vi "stabilizePress_04.vi"() -> ()   [LabVIEW 2011]
uses:
  <vilib>/Platform/TimedLoop/XDataNode/timing_clust.ctl
  <vilib>/Platform/TimedLoop/XDataNode/nitl_modes.ctl
  <vilib>/Platform/TimedLoop/XDataNode/wakeup.ctl
  <vilib>/Platform/TimedLoop/XDataNode/XDataNode.xnode
  <vilib>/Platform/TimedLoop/XDataNode/XDNodeRunTimeDep.lvlib
panel:
  out "tElaps":dbl
  in  "dT_fit(s)":dbl=20.0
  in  "tTotal(s)":dbl=20.0
  out "tNow":dbl
  out "XY Graph":cluster{"Value":dbl[], "Value":dbl[]}(graph)
  out "tune Setpoint(torr)":dbl=20.0
  in  "t array":dbl[](array[numeric])=[1.0, 2.0, 3.0, 4.0, 5.0, 6.0, 7.0, 8.001, 9.0, 10.0, 11.0, 12.0, 13.0, 14.0, 15.0, 16.0, 17.0, 18.001, 19.0, 20.0, 21.0, 22.0]
  out "P array":dbl[](array[numeric])=[20.39, 19.689999999999998, 19.299999999999997, 19.189999999999998, 19.130000000000003, 19.110000000000003, 19.09, 19.08, 19.07, 19.05, 19.04, 19.04, 19.05, 19.05, 19.05, 19.04, 19.05, 19.060000000000002, 19.060000000000002, 19.05, 19.05, 19.05]
  out "stabilize done":bool=TRUE
  in  "tExp(s)":dbl=20.0
  out "Set Point (torr)":dbl=20.0 format="%.2f"
  out "Setpoint Index":string="C"
  out "Setpoint Index control":u16(ring)=2 caption="Setpoint" items=["A", "B", "C", "D"]
  out "first":bool
  out "tStart":dbl=22.0
  in  "time done (s)":dbl
  out "Wait to set":bool
  out "IO error":errorcluster
  in  "stop":bool
  out "P (torr)":dbl=19.05 format="%.2f"
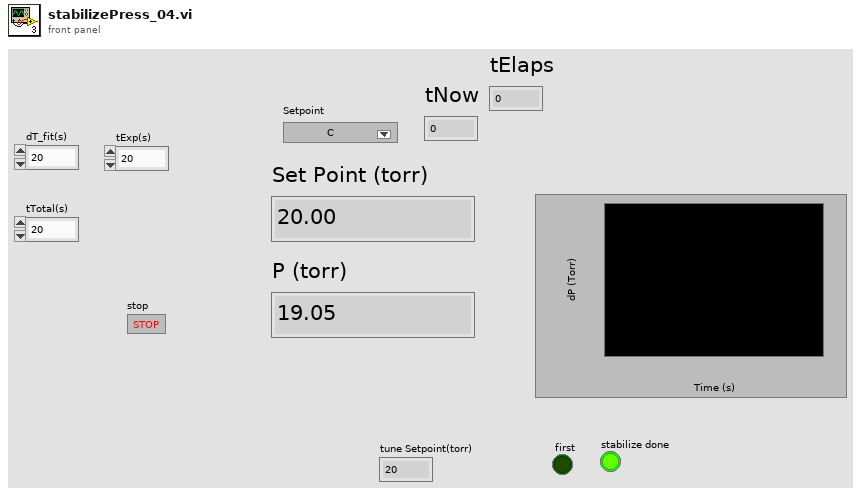
[diagram p1: front panel]
types:
  T1 = typedef "XDNodeRunTimeDep.lvlib/timing_clust.ctl" = cluster{"Expected End [f-1]":u64, "Actual End [f-1]":u64, "Finished Late? [f-1]":bool, "Expected End [i-1]":u64, "Actual End [i-1]":u64, "Finished Late? [i-1]":bool, "Expected Start [i]":u64, "Actual Start [i]":u64, "Expected Start [f]":u64, "Actual Start [f]":u64, "Source Name":string, "Structure Name":string, "Period":i64, "Deadline":i64, "Offset":i64, "Start":i64, "Priority":i32, "Timeout":i32, "Mode":T2, "Wakeup Reason":T3, "Error":errorcluster, "Source Type":string, "Secondary Source Type":string, "Global End Time":u64, "Global Start Time":u64, "Frame Duration":u64, "Iteration Duration":u64, "Assigned CPU":i32, "I/O Scan Engine Mode":u32}
  T2 = typedef "XDNodeRunTimeDep.lvlib/nitl_modes.ctl" = enum32{"No Change", "Process missed periods, maintain original phase", "Discard missed periods, maintain original phase", "Process missed periods, ignore original phase", "Discard missed periods, ignore original phase"}
  T3 = typedef "XDNodeRunTimeDep.lvlib/wakeup.ctl" = enum32{"Normal", "Aborted", "Asynchronous wakeup", "Timing source error", "Timed loop error", "Timeout"}
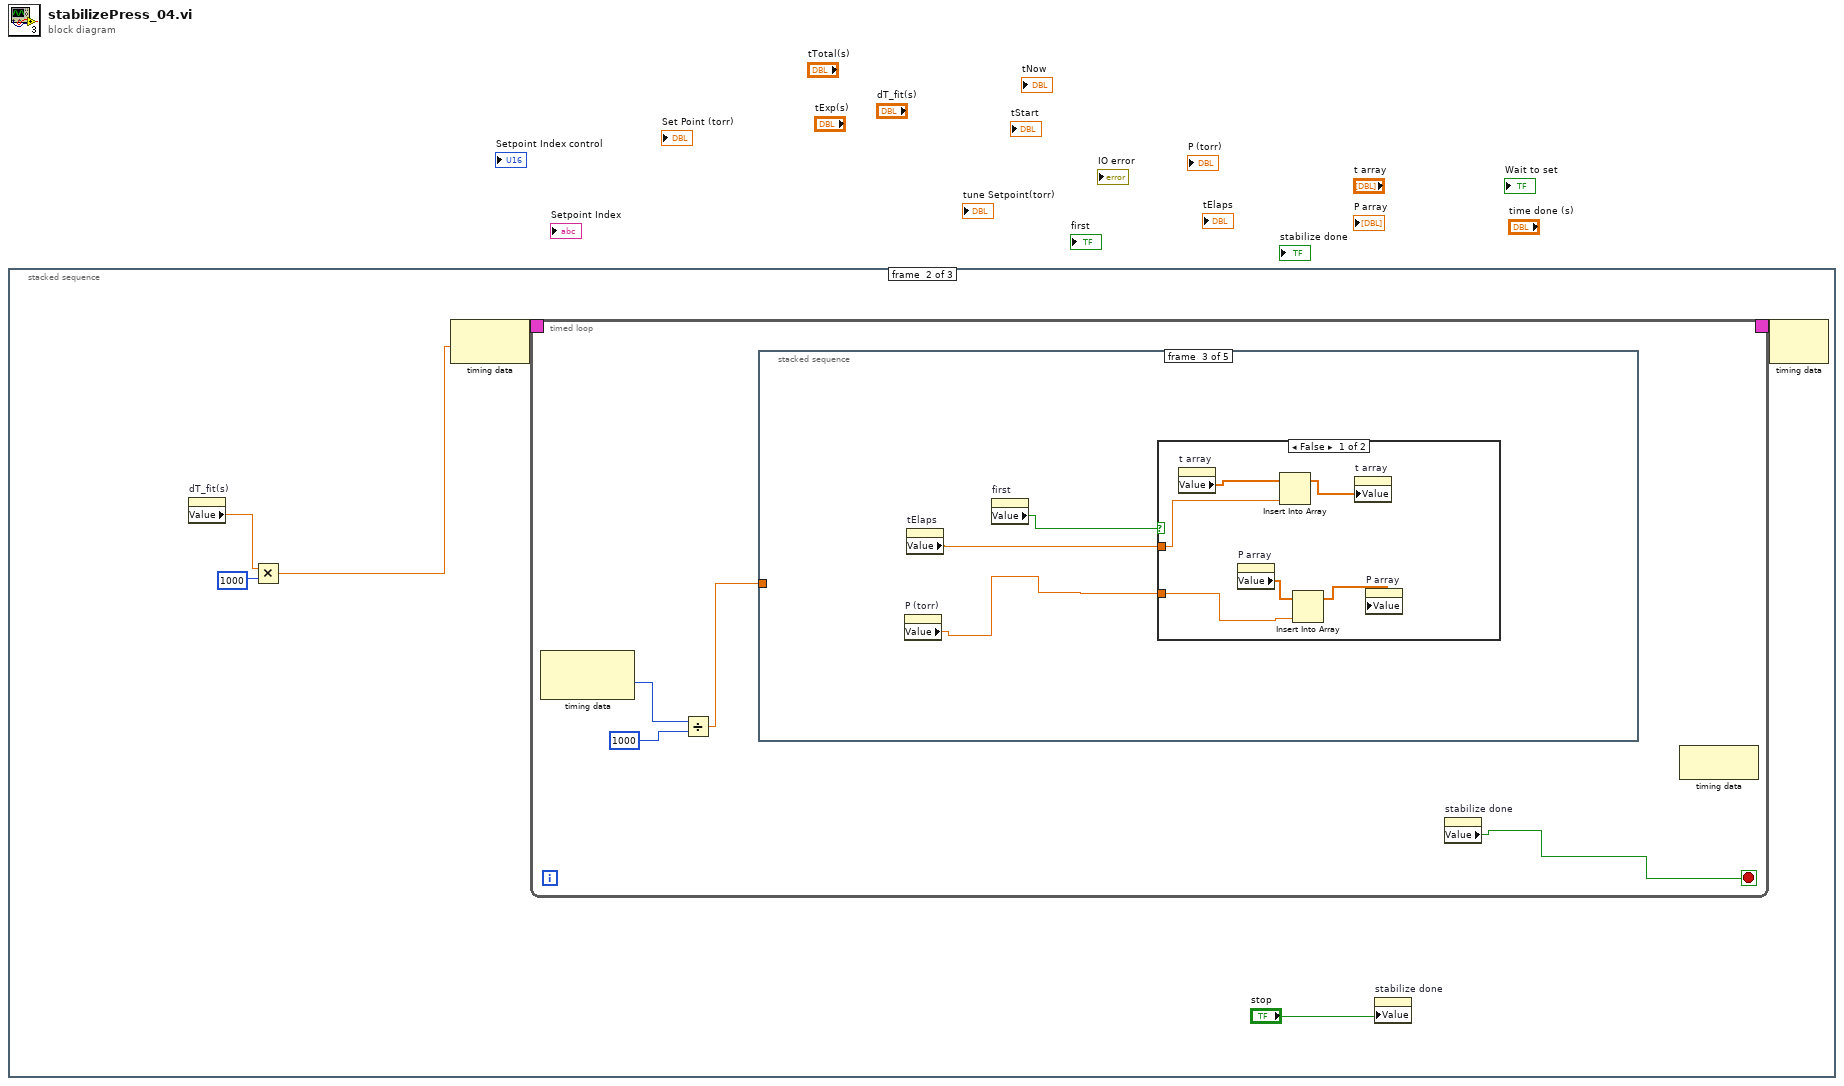
[diagram p0: block diagram]
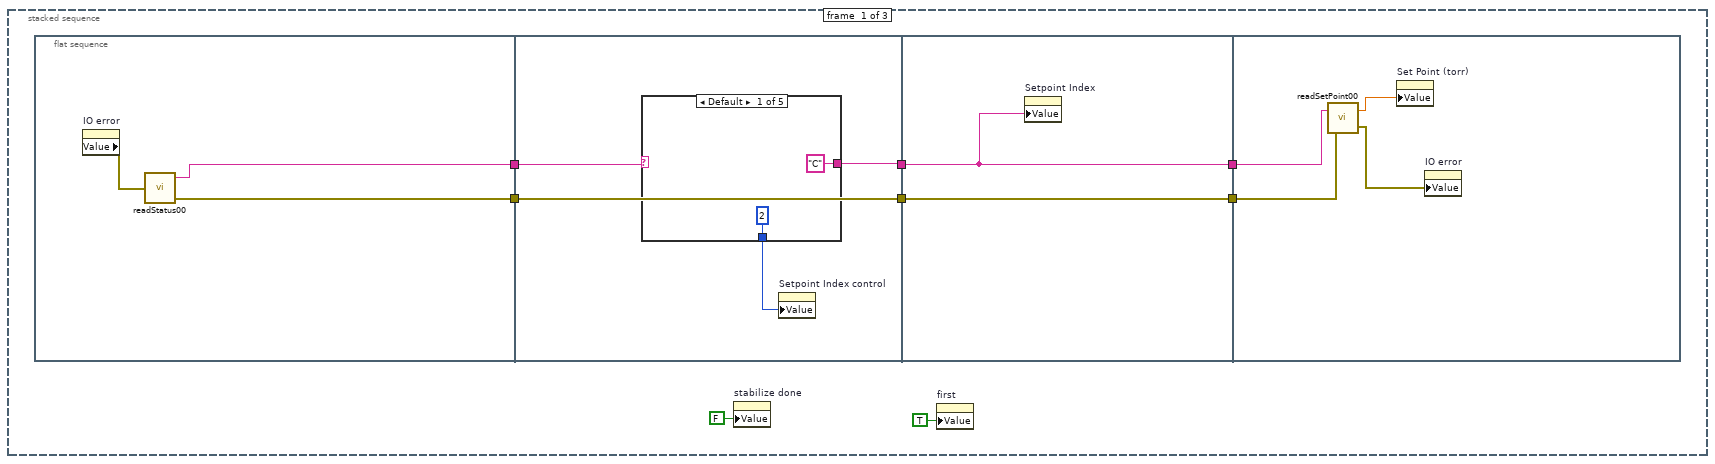
[diagram p2: hidden frame]
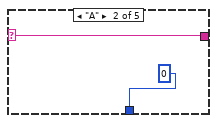
[diagram p3: hidden frame]
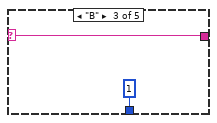
[diagram p4: hidden frame]
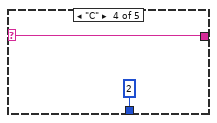
[diagram p5: hidden frame]
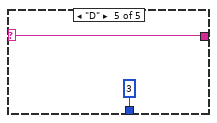
[diagram p6: hidden frame]
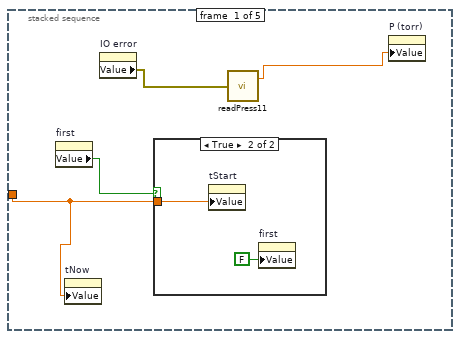
[diagram p7: hidden frame]
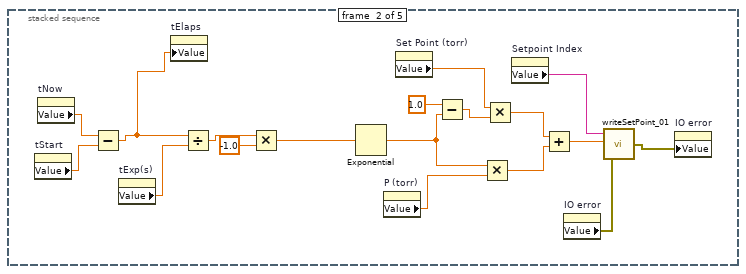
[diagram p9: hidden frame]
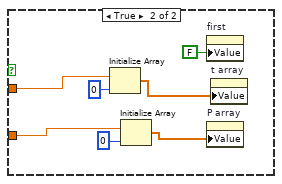
[diagram p10: hidden frame]
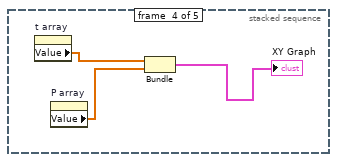
[diagram p11: hidden frame]
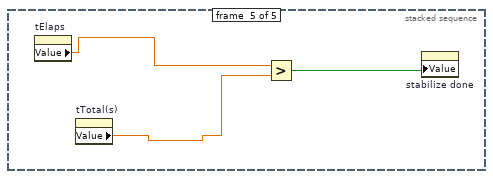
[diagram p12: hidden frame]
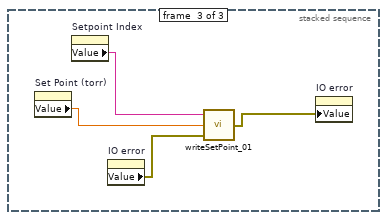
[diagram p13: hidden frame]
diagram:
  n1 = stacked-sequence {
    frame #0 {
      n2 = flat-sequence {
        tunnel: [w10] -> w8
        tunnel: [w9] -> w7
        tunnel: w8 -> [w14]
        tunnel: [w13] -> w6
        tunnel: w7 -> [w15]
        tunnel: [w15] -> w5
        tunnel: w6 -> [w26]
        tunnel: [w26] -> w4
        tunnel: w5 -> [w27]
        tunnel: [w27] -> w3
        tunnel: w4 -> [w31]
        tunnel: w3 -> [w30]
        frame #0 {
          n3 = property on="IO error" class="Clust (strict)"() -> ("Value"=w11:errorcluster)  [unwired: 2 in, 2 out]
          n4 = call "readStatus00.vi"("error in"=w11) -> ("Setpoint"=w10:string, "error out"=w9:errorcluster)  [unwired: 1 out]
        }
        frame #1 {
          n5 = case shown="Default" w14 {
            selector: w14 -> [_ w19 w20 w22 w24]
            tunnel: ["C" w19 w20 w22 w24] -> w13
            tunnel: [u16 2 ("Ring") u16 0 ("Ring") u16 1 ("Ring") u16 2 ("Ring") u16 3 ("Ring")] -> w12
            frame Default {
            }
            frame "A" {
            }
            frame "B" {
            }
            frame "C" {
            }
            frame "D" {
            }
          }
          n6 = property on="Setpoint Index control" class="Ring (strict)"("Value"=w12) -> ()  [unwired: 2 in, 2 out]
        }
        frame #2 {
          n7 = property on="Setpoint Index" class="Str"("Value"=w26) -> ()  [unwired: 2 in, 2 out]
        }
        frame #3 {
          n8 = call "readSetPoint00.vi"("error in"=w30, "Setpoint"=w31) -> ("error out"=w29:errorcluster, "P"=w28:dbl)
          n9 = property on="Set Point (torr)" class="DigNum (strict)"("Value"=w28) -> ()  [unwired: 2 in, 2 out]
          n10 = property on="IO error" class="Clust (strict)"("Value"=w29) -> ()  [unwired: 2 in, 2 out]
        }
      }
      n11 = property on="stabilize done" class="Bool (strict)"("Value"=FALSE ("fit done")) -> ()  [unwired: 2 in, 2 out]
      n12 = property on="first" class="Bool (strict)"("Value"=TRUE ("first")) -> ()  [unwired: 2 in, 2 out]
    }
    frame #1 {
      n13 = property on="dT_fit(s)" class="DigNum (strict)"() -> ("Value"=w33:dbl)  [unwired: 2 in, 2 out]
      n14 = Multiply(x=w33, y=u32 1000) -> (x*y=w34:dbl)
      n15 = node-c288(w34) -> (w37:T1)
      n16 = timed-loop {
        timing: w37 -> [_]
        timing-out: [_] -> w36
        stop <- w38 stop-if-true
        n17 = node-c288() -> (w41:i64)  [unwired: 1 in, 1 out]
        n18 = Divide(x=w41, y=i64 1000) -> (x/y=w39:dbl)
        n19 = stacked-sequence {
          tunnel: w39 -> [w42 _ _ _ _]
          frame #0 {
            n20 = property on="first" class="Bool (strict)"() -> ("Value"=w44:bool)  [unwired: 2 in, 2 out]
            n21 = property on="tNow" class="DigNum (strict)"("Value"=w42) -> ()  [unwired: 2 in, 2 out]
            n22 = property on="IO error" class="Clust (strict)"() -> ("Value"=w45:errorcluster)  [unwired: 2 in, 2 out]
            n23 = case shown="True" w44 {
              tunnel: w42 -> [_ w47]
              frame False {
              }
              frame True {
                n24 = property on="tStart" class="DigNum (strict)"("Value"=w47) -> ()  [unwired: 2 in, 2 out]
                n25 = property on="first" class="Bool (strict)"("Value"=FALSE ("first")) -> ()  [unwired: 2 in, 2 out]
              }
            }
            n26 = call "readPress11.vi"("error in"=w45) -> ("P"=w43:dbl)  [unwired: 1 out]
            n27 = property on="P (torr)" class="DigNum (strict)"("Value"=w43) -> ()  [unwired: 2 in, 2 out]
          }
          frame #1 {
            n28 = property on="tStart" class="DigNum (strict)"() -> ("Value"=w64:dbl)  [unwired: 2 in, 2 out]
            n29 = property on="tNow" class="DigNum (strict)"() -> ("Value"=w65:dbl)  [unwired: 2 in, 2 out]
            n30 = Subtract(x=w65, y=w64) -> (x-y=w48:dbl)
            n31 = property on="tExp(s)" class="DigNum (strict)"() -> ("Value"=w63:dbl)  [unwired: 2 in, 2 out]
            n32 = property on="tElaps" class="DigNum (strict)"("Value"=w48) -> ()  [unwired: 2 in, 2 out]
            n33 = Divide(x=w48, y=w63) -> (x/y=w62:dbl)
            n34 = Multiply(x=w62, y=-1.0) -> (x*y=w60:dbl)
            n35 = Exponential(1:w60) -> (0:w55:dbl)
            n36 = property on="P (torr)" class="DigNum (strict)"() -> ("Value"=w56:dbl)  [unwired: 2 in, 2 out]
            n37 = property on="Set Point (torr)" class="DigNum (strict)"() -> ("Value"=w57:dbl)  [unwired: 2 in, 2 out]
            n38 = Subtract(x=1.0, y=w55) -> (x-y=w58:dbl)
            n39 = Multiply(x=w55, y=w56) -> (x*y=w53:dbl)
            n40 = Multiply(x=w57, y=w58) -> (x*y=w54:dbl)
            n41 = property on="Setpoint Index" class="Str"() -> ("Value"=w51:string)  [unwired: 2 in, 2 out]
            n42 = Add(x=w54, y=w53) -> (x+y=w52:dbl)
            n43 = property on="IO error" class="Clust (strict)"() -> ("Value"=w50:errorcluster)  [unwired: 2 in, 2 out]
            n44 = call "writeSetPoint_01.vi"("error in"=w50, "P (Torr)"=w52, "Setpoint"=w51) -> ("error out"=w49:errorcluster)
            n45 = property on="IO error" class="Clust (strict)"("Value"=w49) -> ()  [unwired: 2 in, 2 out]
          }
          frame #2 {
            n46 = property on="P (torr)" class="DigNum (strict)"() -> ("Value"=w67:dbl)  [unwired: 2 in, 2 out]
            n47 = property on="tElaps" class="DigNum (strict)"() -> ("Value"=w66:dbl)  [unwired: 2 in, 2 out]
            n48 = property on="first" class="Bool (strict)"() -> ("Value"=w68:bool)  [unwired: 2 in, 2 out]
            n49 = case shown="False" w68 {
              tunnel: w67 -> [w74 w80]
              tunnel: w66 -> [w71 w78]
              frame False {
                n50 = property on="t array" class="Arr (strict)"() -> ("Value"=w70:dbl[])  [unwired: 2 in, 2 out]
                n51 = property on="P array" class="Arr (strict)"() -> ("Value"=w72:dbl[])  [unwired: 2 in, 2 out]
                n52 = Insert Into Array(array=w70, new element=w71) -> (w69:dbl[])  [unwired: 1 in]
                n53 = Insert Into Array(array=w72, new element=w74) -> (w73:dbl[])  [unwired: 1 in]
                n54 = property on="t array" class="Arr (strict)"("Value"=w69) -> ()  [unwired: 2 in, 2 out]
                n55 = property on="P array" class="Arr (strict)"("Value"=w73) -> ()  [unwired: 2 in, 2 out]
              }
              frame True {
                n56 = Initialize Array(w78, 0 ("dimension size")) -> (w75:dbl[])
                n57 = Initialize Array(w80, 0 ("dimension size")) -> (w76:dbl[])
                n58 = property on="first" class="Bool (strict)"("Value"=FALSE ("first")) -> ()  [unwired: 2 in, 2 out]
                n59 = property on="P array" class="Arr (strict)"("Value"=w76) -> ()  [unwired: 2 in, 2 out]
                n60 = property on="t array" class="Arr (strict)"("Value"=w75) -> ()  [unwired: 2 in, 2 out]
              }
            }
          }
          frame #3 {
            n61 = property on="t array" class="Arr (strict)"() -> ("Value"=w83:dbl[])  [unwired: 2 in, 2 out]
            n62 = property on="P array" class="Arr (strict)"() -> ("Value"=w84:dbl[])  [unwired: 2 in, 2 out]
            n63 = Bundle "Bundle"("Value"=w83, "Value"=w84) -> (→"XY Graph":cluster{"Value":dbl[], "Value":dbl[]})  [unwired: 1 in]
          }
          frame #4 {
            n64 = property on="tElaps" class="DigNum (strict)"() -> ("Value"=w85:dbl)  [unwired: 2 in, 2 out]
            n65 = property on="tTotal(s)" class="DigNum (strict)"() -> ("Value"=w86:dbl)  [unwired: 2 in, 2 out]
            n66 = Greater?(x=w85, y=w86) -> (0:w87:bool)
            n67 = property on="stabilize done" class="Bool (strict)"("Value"=w87) -> ()  [unwired: 2 in, 2 out]
          }
        }
        n68 = property on="stabilize done" class="Bool (strict)"() -> ("Value"=w38:bool)  [unwired: 2 in, 2 out]
        n69 = node-c288() -> ()  [unwired: 1 in, 1 out]
      }
      n70 = property on="stabilize done" class="Bool (strict)"("Value"="stop") -> ()  [unwired: 2 in, 2 out]
      n71 = node-c288(w36) -> ()  [unwired: 1 out]
    }
    frame #2 {
      n72 = property on="Set Point (torr)" class="DigNum (strict)"() -> ("Value"=w98:dbl)  [unwired: 2 in, 2 out]
      n73 = property on="Setpoint Index" class="Str"() -> ("Value"=w97:string)  [unwired: 2 in, 2 out]
      n74 = property on="IO error" class="Clust (strict)"() -> ("Value"=w96:errorcluster)  [unwired: 2 in, 2 out]
      n75 = call "writeSetPoint_01.vi"("error in"=w96, "P (Torr)"=w98, "Setpoint"=w97) -> ("error out"=w95:errorcluster)
      n76 = property on="IO error" class="Clust (strict)"("Value"=w95) -> ()  [unwired: 2 in, 2 out]
    }
  }
